vi "Configuration Page.vi"(8 "Error in":errorcluster, 11 "INL DNL Test in":refnum<class "INL DNL Test.lvclass">) -> (0 "Error out":errorcluster, 3 "INL DNL Test out":refnum<class "INL DNL Test.lvclass">)   [LabVIEW 2020, in "INL DNL Test.lvclass"]
uses:
  INL DNL Test.lvclass
  D:/SDLC/Class/INL DNL Test/Test/Parent/Test.lvclass
  Typedef/User event controls.ctl
  DNL INL Test.lvlib
panel:
  in  "Best Fit":bool caption="Best Fit method"
  in  "End Point":bool caption="End Point method"
  # "Choose the test method"
  # "Test method"
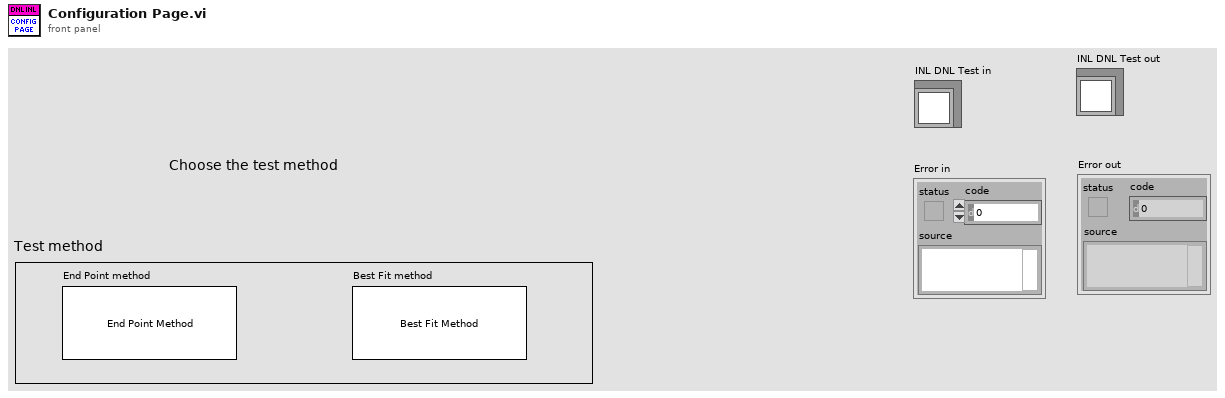
[diagram p1: front panel]
types:
  T1 = typedef "DNL INL Test.lvlib/User event controls.ctl" = enum16{"Create", "Generate", "Run Test", "Get Ref", "Destroy"}
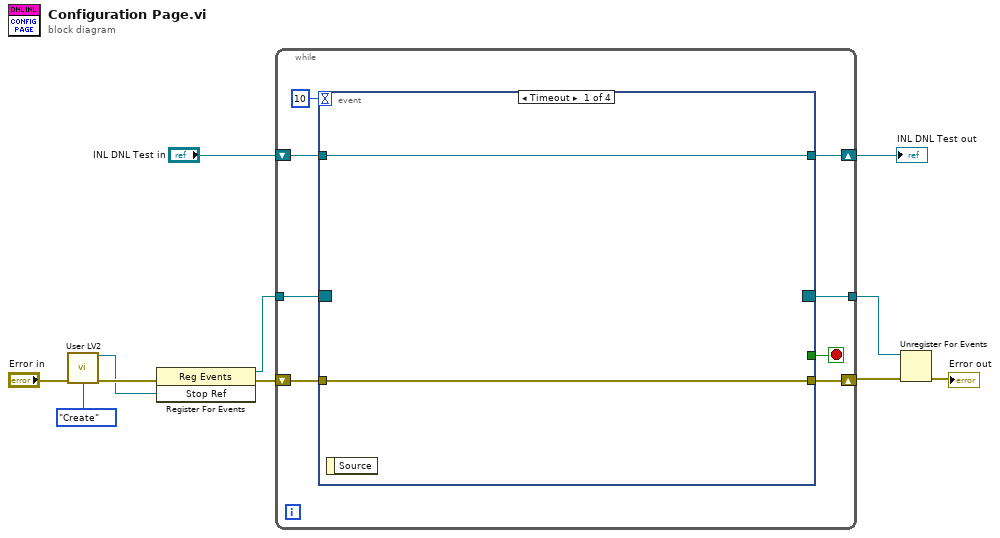
[diagram p0: block diagram]
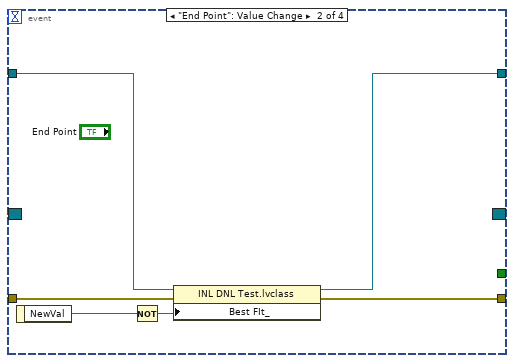
[diagram p2: hidden frame]
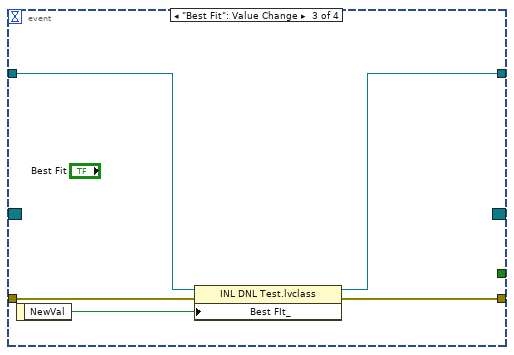
[diagram p3: hidden frame]
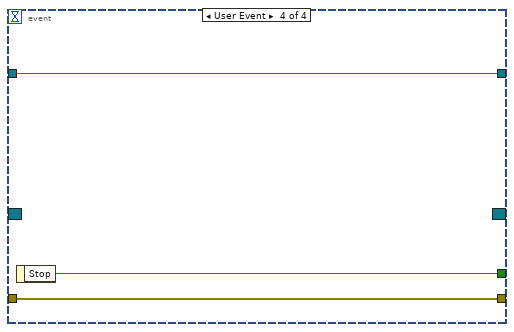
[diagram p4: hidden frame]
diagram:
  n1 = call "User LV2.vi"("Error In"="Error in", "User event controls"=User_event_controls."Create") -> ("Stop Ref"=w8:refnum<user-event>, "Error Out"=w9:errorcluster)  [unwired: 11 in, 1 out]
  n2 = register-events(error in=w9, w8) -> (reference out=w7:refnum<event-registration>, error out=w4:errorcluster)  [unwired: 1 in]
  n3 = while {
    tunnel: w7 -> [w19]
    shift-right: [w16] -> w5
    shift-left: "INL DNL Test in" -> [w17]
    shift-right: [w13] -> w2
    shift-left: w4 -> [w14]
    tunnel: [w12] -> w1
    stop <- w15 stop-if-true
    n4 = event shown="[0] Timeout" {
      selector: w19 -> [_ _ _ _]
      dyn-events: [_ _ _ _] -> w12
      timeout: 10 -> [_ _ _ _]
      tunnel: [w20 w23 w29 w33] -> w16
      tunnel: w17 -> [w20 w26 w31 w33]
      tunnel: [_ _ _ w35] -> w15
      tunnel: w14 -> [w21 w27 w32 w34]
      tunnel: [w21 w22 w30 w34] -> w13
      event Timeout {
        n5 = event-data() -> ()  [unwired: 1 in, 1 out]
      }
      event "End Point": Value Change {
        n6 = event-data() -> ("NewVal"=w25:bool)  [unwired: 1 in]
        n7 = Not(x=w25) -> (.not. x?=w24:bool)
        n8 = property class="INL DNL Test.lvclass"(reference=w26, error in=w27, "Best FIt_"=w24) -> (reference out=w23:refnum<class "INL DNL Test.lvclass">, error out=w22:errorcluster)
      }
      event "Best Fit": Value Change {
        n9 = event-data() -> ("NewVal"=w28:bool)  [unwired: 1 in]
        n10 = property class="INL DNL Test.lvclass"(reference=w31, error in=w32, "Best FIt_"=w28) -> (reference out=w29:refnum<class "INL DNL Test.lvclass">, error out=w30:errorcluster)
      }
      event User Event {
        n11 = event-data() -> ("Stop"=w35:bool)  [unwired: 1 in]
      }
    }
  }
  "INL DNL Test out" <- w5
  n12 = Unregister For Events(event registration refnum=w1, error in=w2) -> (error out=→"Error out":errorcluster)
